vi "BioFeedback4(AudioInput+ModularDesign).vi"() -> ()   [LabVIEW 2016]
uses:
  Control 2.ctl
  <vilib>/Analysis/5stat.llb/RMS (DBL).vi
  <vilib>/Analysis/NI_AALPro.lvlib
panel:
  in  "Trial":dbl
  out "(INTERNAL) Buffer Array Size":i32
  out "(INTERNAL) Buffer Index":i32
  out "smooth":dynamicdata(graph)
  out "Thermometer Elapsed Frames":i32
  in  "Thermometer\nFps":dbl
  out "AggregateSignalData":waveform(dbl)[](array[waveform])
  out "rms data":dbl(graph)
  in  "Start":bool
  out "Data Levels":dbl(slide) scale=0.0..0.07
  out "Moving Average Length (s)":dbl
  in  "Sample rate (Hz)":dbl=22050.0
  in  "Sample Duration (s)":T1=0.1 caption="Duration (s)"
  in  "Stop Recording":bool
  in  "Lower Cut-Off (Hz)":dbl=20.0 caption="Lower Cut-Off"
  in  "Upper Cut-Off (Hz)":dbl=300.0 caption="Upper Cut-Off"
  out "filtered signal (single sample)":waveform(dbl)(graph)
  out "aggregate signal":waveform(dbl)[](graph)
  in  "Number of Samples in\n Moving Average":dbl
  # "Biofeedback"
  # "Internal"
  # "Settings"
  # "Filter Settings"
  # "Bandpass Filter"
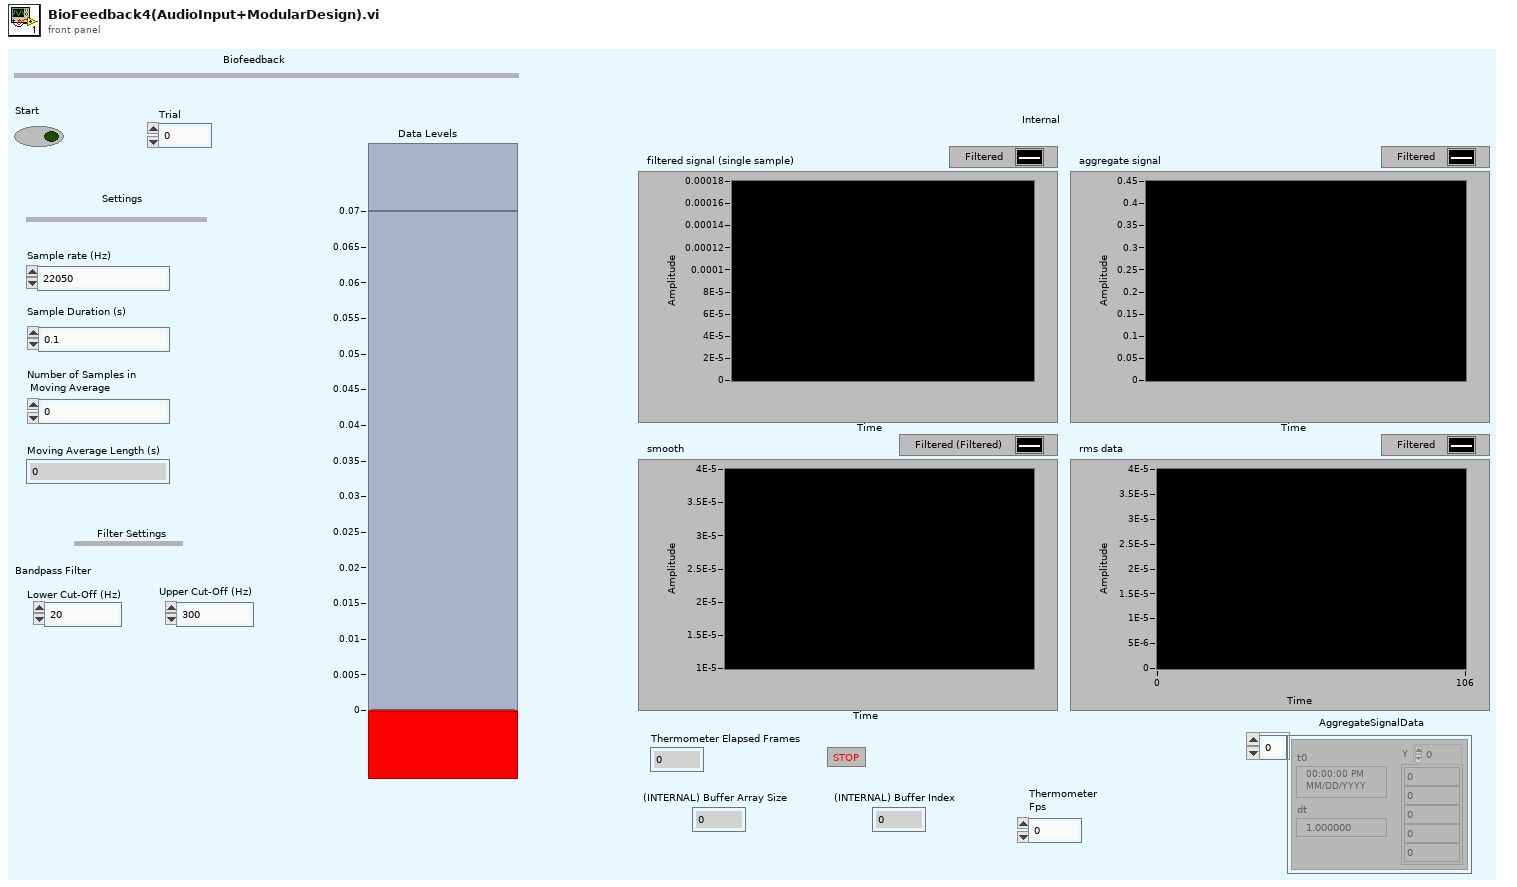
[diagram p1: front panel]
types:
  T1 = typedef "Control 2.ctl" = dbl
  T2 = typedef "WaveformArrayControl.ctl" = waveform(dbl)[]
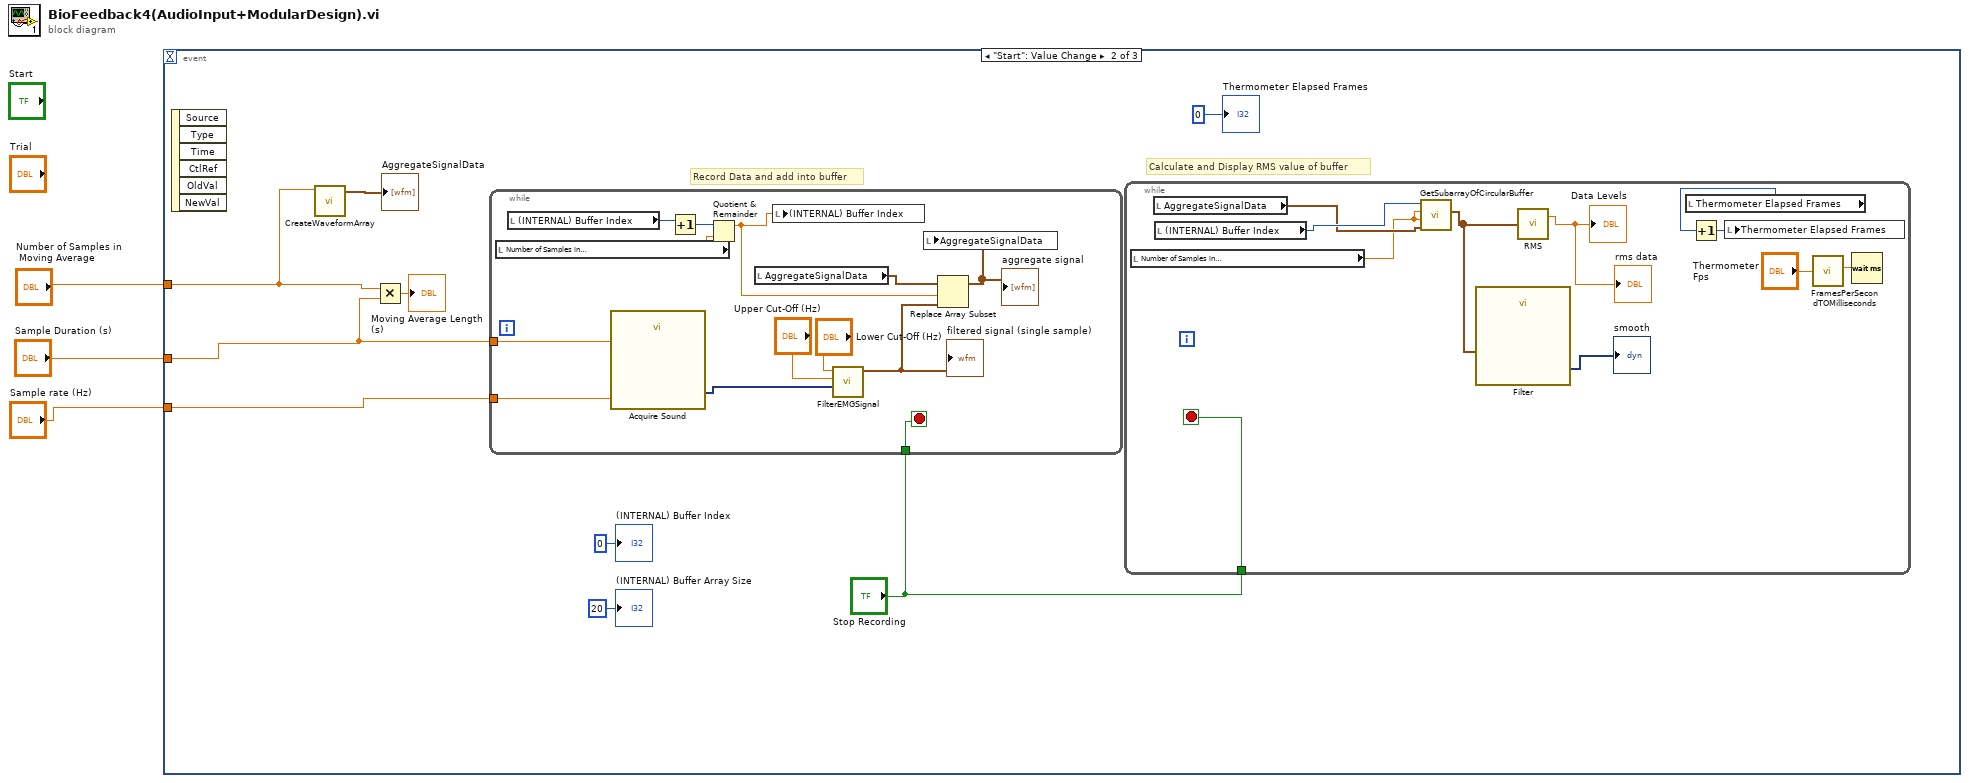
[diagram p0: block diagram]
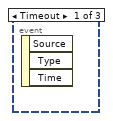
[diagram p2: hidden frame]
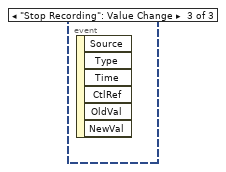
[diagram p3: hidden frame]
diagram:
  n1 = event shown="[1] \"Start\": Value Change" {
    selector: _ -> [_ _ _]
    dyn-events: _ -> [_ _ _]
    timeout: _ -> [_ _ _]
    tunnel: "Number of Samples in\n Moving Average" -> [_ w7 _]
    tunnel: "Sample Duration (s)" -> [_ w6 _]
    tunnel: "Sample rate (Hz)" -> [_ w5 _]
    event Timeout {
      n2 = event-data() -> ()  [unwired: 1 in, 3 out]
    }
    event "Start": Value Change {
      # "Record Data and add into buffer"
      # "Calculate and Display RMS value of buffer"
      n3 = event-data() -> ()  [unwired: 1 in, 6 out]
      n4 = call "CreateWaveformArray.vi"("bufferSize"=w7) -> ("initialized array"=→"AggregateSignalData":waveform(dbl)[])  [unwired: 10 in]
      n5 = Multiply(x=w7, y=w6) -> (x*y=→"Moving Average Length (s)":T1)
      n6 = while {
        tunnel: "Stop Recording" -> [w34]
        tunnel: w6 -> [w33]
        tunnel: w5 -> [w32]
        stop <- w34 stop-if-true
        n7 = local read "Number of Samples in\n Moving Average"() -> (w26:dbl)
        n8 = local read "(INTERNAL) Buffer Index"() -> (w28:i32)
        n9 = call "Acquire Sound"("Duration (s)"=w33, "Sample rate (Hz)"=w32) -> ("Data"=w25:dynamicdata)  [unwired: 16 in, 1 out]
        n10 = Increment(x=w28) -> (x+1=w27:i32)
        n11 = Quotient & Remainder(x=w27, y=w26) -> (x-y*floor(x/y)=w24:dbl)  [unwired: 1 out]
        n12 = local read "AggregateSignalData"() -> (w30:waveform(dbl)[])
        n13 = local write "(INTERNAL) Buffer Index"(w24) -> ()
        n14 = call "FilterEMGSignal.vi"("Data"=w25, "Upper Cut-Off"="Upper Cut-Off (Hz)", "Lower Cut-Off"="Lower Cut-Off (Hz)") -> ("Waveform"=w31:waveform(dbl))  [unwired: 8 in]
        "filtered signal (single sample)" <- w31
        n15 = Replace Array Subset(array=w30, new element=w31, index=w24) -> (w29:waveform(dbl)[])
        "aggregate signal" <- w29
        n16 = local write "AggregateSignalData"(w29) -> ()
      }
      n17 = while {
        tunnel: "Stop Recording" -> [w23]
        stop <- w23 stop-if-true
        n18 = local read "Number of Samples in\n Moving Average"() -> (w13:dbl)
        n19 = local read "AggregateSignalData"() -> (w16:waveform(dbl)[])
        n20 = local read "(INTERNAL) Buffer Index"() -> (w17:i32)
        n21 = call "GetSubarrayOfCircularBuffer.vi"("initialized array"=w16, "buffer size"=w13, "subset size"=w13, "start index"=w17) -> ("initialized array 2"=w15:T2)  [unwired: 7 in]
        n22 = call "Filter"("Signal"=w15) -> ("Filtered Signal"=→"smooth":dynamicdata)  [unwired: 9 in, 1 out]
        n23 = call-poly <vilib>:"RMS.vi"("X"=w15) -> ("rms value"=→"Data Levels" →"rms data":dbl)  [unwired: 1 out]
        n24 = local read "Thermometer Elapsed Frames"() -> (w20:i32)
        n25 = Increment(x=w20) -> (x+1=w19:i32)
        n26 = local write "Thermometer Elapsed Frames"(w19) -> ()
        n27 = call "FramesPerSecondTOMilliseconds.vi"("Thermometer\nFps"="Thermometer\nFps") -> ("x*y"=w21:dbl)  [unwired: 10 in]
        n28 = Wait (ms)(milliseconds to wait=w21) -> ()  [unwired: 1 out]
      }
      "Thermometer Elapsed Frames" <- 0 ("Thermometer Elapsed Frames")
      "(INTERNAL) Buffer Index" <- 0 ("Current Buffer Index")
      "(INTERNAL) Buffer Array Size" <- 20 ("(INTERNAL) Buffer Array Size")
    }
    event "Stop Recording": Value Change {
      n29 = event-data() -> ()  [unwired: 1 in, 6 out]
    }
  }
